vi "BuildEXE.vi"(5 "Wait for debugger on launch (false)":bool, 6 "VersionString":string="v1.2.3", 7 "Enable debugging (false)":bool, 8 "error in":errorcluster, 9 "DestinationDir":path=path "C:/Users/pauloneill/SCC/Orion/LabVIEW/Builds/Orion", 10 "BuildSpec":string="Orion", 11 "ProjectPath":path=path "C:/Users/pauloneill/SCC/Orion/LabVIEW/Source/App/Orion.lvproj") -> (0 "error out":errorcluster, 3 "GeneratedFiles":path[](array[path]))   [LabVIEW 2020, in "CICD.lvlib"]
uses:
  CICD.lvlib
  <vilib>/AppBuilder/AB_API/EXE/NI_AB_API_EXE.lvclass
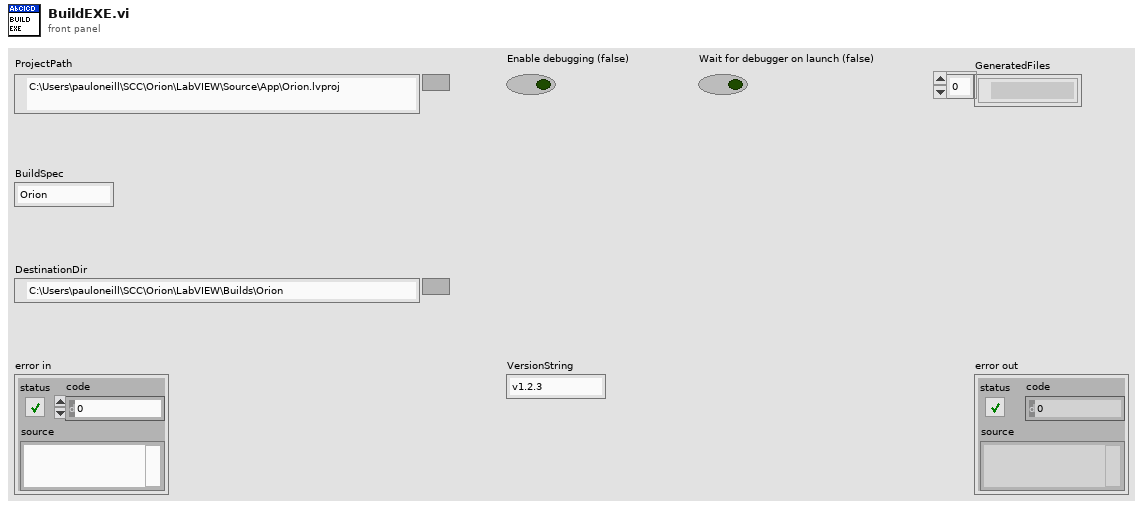
[diagram p1: front panel]
types:
  T1 = typedef "NI_App_Builder_API.lvlib/Build Specification Version.ctl" = cluster{"Major":u16, "Minor":u16, "Fix":u16, "Build":u16}
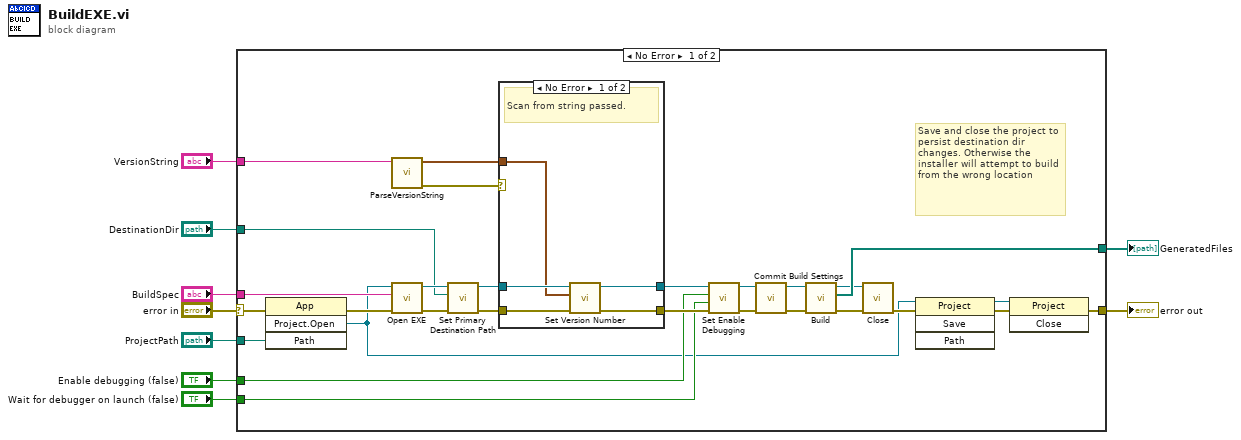
[diagram p0: block diagram]
diagram:
  n1 = case shown="No Error" "error in" {
    selector: "error in" -> [w15 w45]
    tunnel: [w11 w45] -> w9
    tunnel: "VersionString" -> [w30 _]
    tunnel: [w29 _] -> w6
    tunnel: "DestinationDir" -> [w24 _]
    tunnel: "BuildSpec" -> [w26 _]
    tunnel: "ProjectPath" -> [w27 _]
    tunnel: "Enable debugging (false)" -> [w21 _]
    tunnel: "Wait for debugger on launch (false)" -> [w20 _]
    frame No Error {
      # "Save and close the project to persist destination dir changes. Otherwise the installer will attempt to build from the wrong location"
      n2 = invoke class="App" method="Project.Open"(error in=w15, "Path"=w27) -> (error out=w14:errorcluster, "Project:Open"=w13:refnum<vi>)  [unwired: 2 in, 2 out]
      n3 = call "ParseVersionString.vi"("VersionString"=w30) -> ("error out"=w37:errorcluster, "Build spec version"=w31:T1)  [unwired: 9 in]
      n4 = call <vilib>:"Open EXE.vi"("error in (no error)"=w14, "Build specification name"=w26, "Project Refnum"=w13) -> ("error out"=w34:errorcluster, "EXE out"=w25:refnum<class "NI_AB_API_EXE.lvclass">)  [unwired: 7 in]
      n5 = call-dynamic "Set Primary Destination Path.vi"("error in (no error)"=w34, "Destination path"=w24, "Build in"=w25) -> ("error out"=w33:errorcluster, "Build out"=w23:refnum<class "NI_AB_API_EXE.lvclass">)  [unwired: 7 in]
      n6 = case shown="No Error" w37 {
        tunnel: [w41 w43] -> w22
        tunnel: [w42 w44] -> w32
        tunnel: w23 -> [w39 w43]
        tunnel: w33 -> [w40 w44]
        tunnel: w31 -> [w38 _]
        frame No Error {
          # "Scan from string passed."
          n7 = call-dynamic "Set Version Number.vi"("error in (no error)"=w40, "Version number"=w38, "EXE in"=w39) -> ("error out"=w42:errorcluster, "EXE out"=w41:refnum<class "NI_AB_API_EXE.lvclass">)  [unwired: 7 in]
        }
        frame Error {
          # "Could not parse version string - leave as is."
        }
      }
      n8 = call-dynamic "Set Enable Debugging.vi"("error in (no error)"=w32, "Wait for debugger on launch (false)"=w20, "Enable debugging (false)"=w21, "EXE in"=w22) -> ("error out"=w17:errorcluster, "EXE out"=w19:refnum<class "NI_AB_API_EXE.lvclass">)  [unwired: 6 in]
      n9 = call-dynamic "Commit Build Settings.vi"("error in (no error)"=w17, "EXE in"=w19) -> ("error out"=w16:errorcluster, "EXE out"=w18:refnum<class "NI_AB_API_EXE.lvclass">)  [unwired: 8 in]
      n10 = call-dynamic "Build.vi"("error in (no error)"=w16, "EXE in"=w18) -> ("error out"=w36:errorcluster, "GeneratedFiles"=w29:path[], "EXE out"=w28:refnum<class "NI_AB_API_EXE.lvclass">)  [unwired: 6 in, 1 out]
      n11 = call-dynamic "Close.vi"("error in (no error)"=w36, "EXE in"=w28) -> ("error out"=w35:errorcluster)  [unwired: 9 in]
      n12 = invoke class="Project" method="Save"(reference=w13, error in=w35) -> (reference out=w10:refnum<vi>, error out=w12:errorcluster)  [unwired: 2 in, 2 out]
      n13 = invoke class="Project" method="Close"(reference=w10, error in=w12) -> (error out=w11:errorcluster)  [unwired: 1 in, 2 out]
    }
    frame Error {
    }
  }
  "GeneratedFiles" <- w6
  "error out" <- w9
